vi "GetData.vi"(8 "error in (no error)":errorcluster, 11 "MsgPackSerializer in":refnum<class "MsgPackSerializer.lvclass">) -> (0 "error out":errorcluster, 3 "Data":string)   [LabVIEW 2015, in "MsgPackSerializer.lvclass"]
uses:
  MsgPackSerializer.lvclass
  MsgPackSerializer.lvclass/MsgPackSerializer.ctl
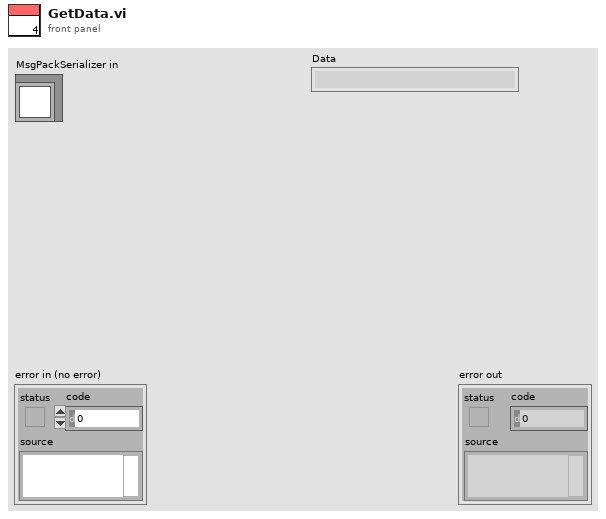
[diagram p1: front panel]
types:
  T1 = typedef "MsgPackSerializer.lvclass/Fragment.ctl" = cluster{"DVR":refnum<data-value>, "Length":i64}
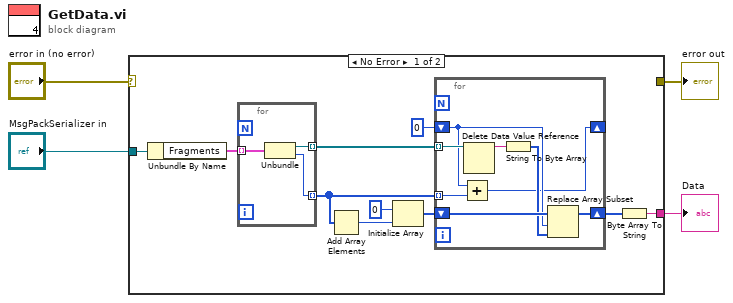
[diagram p0: block diagram]
diagram:
  n1 = case shown="No Error" "error in (no error)" {
    selector: "error in (no error)" -> [_ w26]
    tunnel: [_ w26] -> w3
    tunnel: "MsgPackSerializer in" -> [w14 _]
    tunnel: [w7 _] -> w1
    frame No Error {
      n2 = Unbundle By Name(w14) -> ("Fragments"=w13:T1[])
      n3 = for {
        tunnel: w13 -> [w25] mode=indexing
        tunnel: [w24] -> w9 mode=indexing
        tunnel: [w23] -> w6 mode=indexing
        n4 = Unbundle(w25) -> ("DVR"=w23:refnum<data-value>, "Length"=w24:i64)
      }
      n5 = Add Array Elements(numeric array=w9) -> (sum=w12:i64)
      n6 = Initialize Array(u8 0 ("element"), w12) -> (w10:u8[])
      n7 = for {
        shift-right: [w21] -> w8
        shift-left: w10 -> [w22]
        tunnel: w9 -> [w16] mode=indexing
        tunnel: w6 -> [w19] mode=indexing
        shift-right: [w15] -> _
        shift-left: u8 0 ("element") -> [w17]
        n8 = Add(x=w17, y=w16) -> (x+y=w15:i64)
        n9 = Delete Data Value Reference(data value reference=w19) -> (data value=w20:string)  [unwired: 1 in, 1 out]
        n10 = String To Byte Array(string=w20) -> (unsigned byte array=w18:u8[])
        n11 = Replace Array Subset(array=w22, new element=w18, index=w17) -> (w21:u8[])
      }
      n12 = Byte Array To String(unsigned byte array=w8) -> (string=w7:string)
    }
    frame Error {
    }
  }
  "error out" <- w3
  "Data" <- w1
